vi "Query Page VI Path.vi"(7 "searching path":path[](array[path]), 8 "Error in":errorcluster caption="Error in (no error)", 11 "page name":string="-") -> (0 "Error out":errorcluster, 3 "path":path)   [LabVIEW 2020, in "CSM-TagDBDisplayWnd.lvlib"]
uses:
  CSM-TagDBDisplayWnd.lvlib
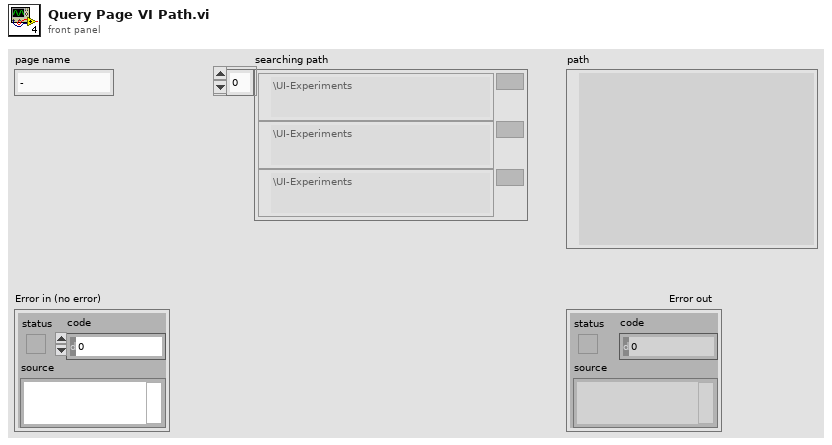
[diagram p1: front panel]
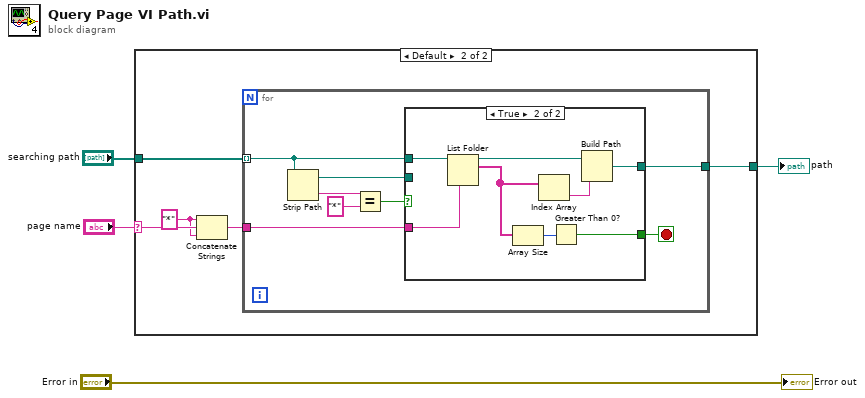
[diagram p0: block diagram]
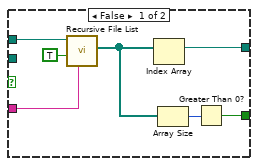
[diagram p3: hidden frame]
diagram:
  n1 = case shown="Default" "page name" {
    selector: "page name" -> [_ w8]
    tunnel: "searching path" -> [_ w9]
    tunnel: [_ w5] -> w2
    frame "" {
    }
    frame Default {
      w7 = "*" ("string")
      n2 = Concatenate Strings(w7, w8, w7) -> (w6:string)
      n3 = for {
        tunnel: w9 -> [w16] mode=indexing
        tunnel: w6 -> [w17]
        tunnel: [w10] -> w5
        stop <- w11 stop-if-true
        n4 = Strip Path(path=w16) -> (stripped path=w12:path, name=w15:string)
        n5 = Equal?(x=w15, y="*") -> (x = y?=w13:bool)
        n6 = case shown="True" w13 {
          tunnel: w17 -> [w24 w32]
          tunnel: [w20 w25] -> w10
          tunnel: w16 -> [w23 w31]
          tunnel: w12 -> [_ _]
          tunnel: [w18 w26] -> w11
          frame False {
            n7 = call <vilib>:"Recursive File List.vi"("pattern"=w24, "Continue Recursing on Error? (F)"=TRUE, "Folder Path"=w23) -> ("All Files in Dir"=w19:path[])  [unwired: 4 in, 4 out]
            n8 = Index Array(array=w19) -> (element=w20:path)  [unwired: 1 in]
            n9 = Array Size(array=w19) -> (size(s)=w21:i32)
            n10 = Greater Than 0?(x=w21) -> (x > 0?=w18:bool)
          }
          frame True {
            n11 = List Folder(path=w31, pattern=w32) -> (path out=w27:path, filenames=w28:string[])  [unwired: 2 in, 2 out]
            n12 = Array Size(array=w28) -> (size(s)=w30:i32)
            n13 = Index Array(array=w28) -> (element=w29:string)  [unwired: 1 in]
            n14 = Greater Than 0?(x=w30) -> (x > 0?=w26:bool)
            n15 = Build Path(base path=w27, name or relative path=w29) -> (appended path=w25:path)
          }
        }
      }
    }
  }
  "path" <- w2
  "Error out" <- "Error in"
